vi "Write Data.vi"(8 "error in (no error)":errorcluster, 10 "Data":sgl[](array[numeric]), 11 "Single_Array in":refnum<class "Single_Array.lvclass">) -> (0 "error out":errorcluster, 3 "Single_Array out":refnum<class "Single_Array.lvclass">)   [LabVIEW 2012, in "Base Data Class.lvlib" / "Single_Array.lvclass"]
uses:
  Single_Array.lvclass
  Single_Array.lvclass/Single_Array.ctl
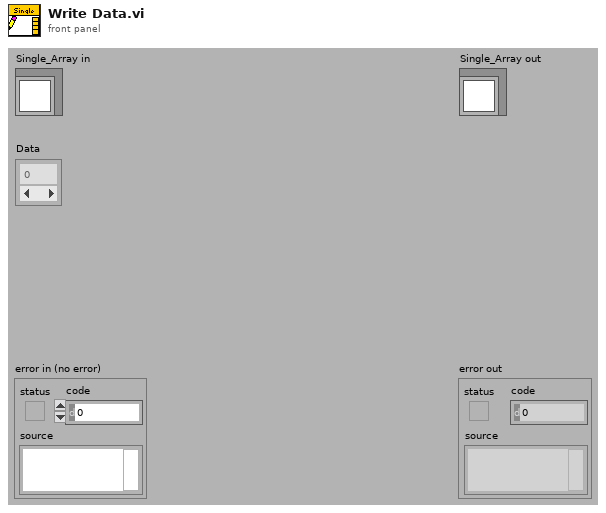
[diagram p1: front panel]
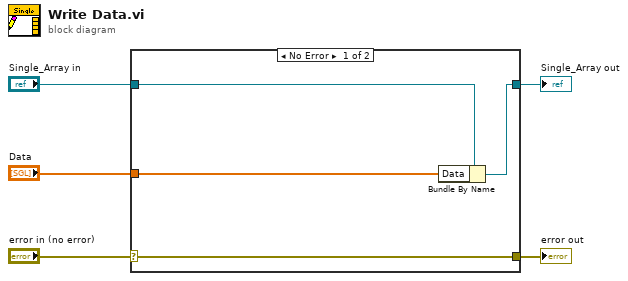
[diagram p0: block diagram]
diagram:
  n1 = case shown="No Error" "error in (no error)" {
    selector: "error in (no error)" -> [w9 w10]
    tunnel: [w9 w10] -> w4
    tunnel: [w7 w11] -> w2
    tunnel: "Single_Array in" -> [w8 w11]
    tunnel: "Data" -> [w6 _]
    frame No Error {
      n2 = Bundle By Name(cluster=w8, "Data"=w6) -> (w7:refnum<class "Single_Array.lvclass">)
    }
    frame Error {
    }
  }
  "error out" <- w4
  "Single_Array out" <- w2
